vi "Read l (nm).vi"(8 "error in":errorcluster, 11 "PAS Cell in":refnum<class "PAS Cell.lvclass">) -> (0 "error out":errorcluster, 2 "l (nm)":T1, 3 "PAS Cell out":refnum<class "PAS Cell.lvclass">)   [LabVIEW 2015, in "PAS Cell.lvclass"]
uses:
  PAS Cell.lvclass
  Main/Controls/LasLam.ctl
  PAS Cell.lvclass/PAS Cell.ctl
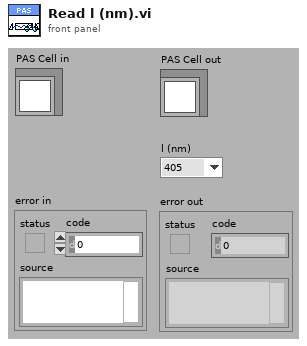
[diagram p1: front panel]
types:
  T1 = typedef "LasLam.ctl" = enum16{"405", "532", "661"}
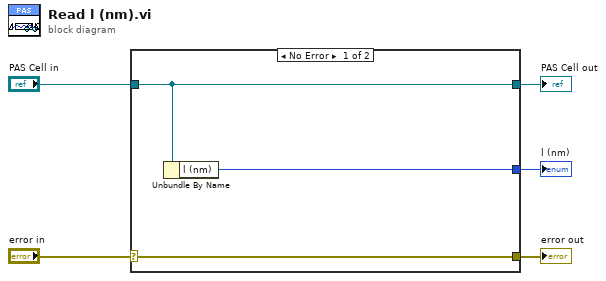
[diagram p0: block diagram]
diagram:
  n1 = case shown="No Error" "error in" {
    selector: "error in" -> [w8 w9]
    tunnel: [w8 w9] -> w4
    tunnel: [w7 w10] -> w2
    tunnel: "PAS Cell in" -> [w7 w10]
    tunnel: [w6 _] -> w1
    frame No Error {
      n2 = Unbundle By Name(w7) -> ("l (nm)"=w6:T1)
    }
    frame Error {
    }
  }
  "error out" <- w4
  "PAS Cell out" <- w2
  "l (nm)" <- w1
